vi "DataLog Databases Module.vi"(5 "LuaVIEW reference":T1, 7 "function index":i32) -> (15 "error out":errorcluster)   [LabVIEW 2012]
doc: "Module required by the \"databases\" runlevel. It enumerates the logging databases by scanning their directories and instantiates in-memory objects reflecting the tags in each database. Performs recovery of aggregated log data if needed. Exports tag management and query functions."
uses:
  luaview/typedefs/t_LuaVIEW Reference.ctl
  typedefs/t_DataLog Databases Methods.ctl
  typedefs/t_Datalog Datebase Modes.ctl
  typedefs/t_DataLog Tag Info List Methods.ctl
  luaview/subvis/private/LuaVIEW Pull (string).vi
  luaview/subvis/private/LuaVIEW Pull (refnum).vi
  subvis/private/glb_DataLog Runtime Parameterisation.vi
  luaview/subvis/private/LuaVIEW Pull (flat data).vi
  luaview/subvis/private/LuaVIEW Push (object).vi
  luaview/subvis/private/LuaVIEW Push (string).vi
  subvis/private/glb_DataLog MCVD.vi
  luaview/subvis/private/LuaVIEW Pull (number).vi
  luaview/subvis/private/LuaVIEW Push (boolean).vi
  luaview/subvis/private/LuaVIEW Push (flat data).vi
  luaview/subvis/private/LuaVIEW Push (number).vi
  luaview/subvis/private/LuaVIEW Push (I32).vi
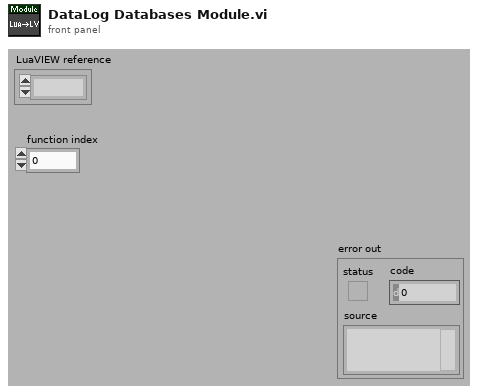
[diagram p1: front panel]
types:
  T1 = typedef "t_LuaVIEW Reference.ctl" = refnum<k1>
  T2 = enum32{"initialize", "init config", "init check config", "init recover", "init error?", "!DB.lookup([str:name])", "!DB.create(obj:db,str:tag,tab:config,[any:initial])", "!DB.delete(obj:db,str:tag)", "!bool:exists=DB.exists(obj:db,str:tag)", "!tab:config=DB.config(obj:db,str:tag)", "!tab:tags=DB.list(obj:db,[str:pattern])", "!any:value,num:time=DB.last(obj:db,str:tag)", "!num:values=DB.logsize(obj:db,str:tag)", "!str:mode=DB.mode(obj:db)", "!DB.reconfigure(obj:db,str:tag,tab:config)", "!tab:tags=DB.subset(obj:db,str:subset)", "!tab:subsets=DB.subsets(obj:db)", "!num:tags=DB.tags(obj:db)", "!str:basetag=stripmeta(str:metatag)", "revoke_exports()", "cleanup()"}
  T3 = typedef "t_DataLog Databases Methods.ctl" = enum16{"initialize", "get ref", "get names", "cleanup"}
  T4 = typedef "t_DataLog Tag Info List Methods.ctl" = enum16{"initialize", "create", "create empty", "rename", "delete", "test tag", "get", "get by name", "get default", "get list", "get path", "get subsets", "set subsets", "set config", "set capacity", "#tags", "go live", "set unlocked", "set mirrored"}
  T5 = typedef "t_Datalog Datebase Modes.ctl" = enum16{"locked", "unlocked", "live", "mirrored"}
  T6 = cluster{"databases":cluster{"mode":T5, "path":path}[], "recovery directory":path, "max points":i32, "max string mem":i32}
  T7 = typedef "t_DataLog Database Info Pane.ctl" = refnum<vi>
  T8 = typedef "t_DataLog Tag Config.ctl" = cluster{"name":string, "unit":string, "temporal":T9, "value":T10, "index":i32, "capacity":i32, "is meta?":bool, "mincapacity":i32, "deadband":dbl, "limit delay":dbl, "format":T11, "precision":u8, "undefine":bool, "update":bool, "update period":u16, "expression":string, "description":string, "logging algorithm":T12, "logging parameters":dbl[]}
  T9 = typedef "t_DataLog Temporal Types.ctl" = enum16{"set&hold", "sample", "event"}
  T10 = typedef "t_DataLog Value Types.ctl" = enum16{"number", "string"}
  T11 = typedef "t_DataLog Numerical Format.ctl" = enum8{"fractional", "exponential", "engineering"}
  T12 = typedef "t_DataLog Logging Algorithms.ctl" = enum16{"nothing", "changes", "everything", "every Nth", "time threshold", "value threshold + prior", "t or v threshold", "t or v threshold + prior"}
  T13 = typedef "et_DataLog Meta Tag Specifier.ctl" = enum32{"warn_lo", "warn_hi", "A_lo", "A_hi", "B_lo", "B_hi", "C_lo", "C_hi", "D_lo", "D_hi", "E_lo", "E_hi", "F_lo", "F_hi", "G_lo", "G_hi", "H_lo", "H_hi", "I_lo", "I_hi", "J_lo", "J_hi", "K_lo", "K_hi", "L_lo", "L_hi", "M_lo", "M_hi", "N_lo", "N_hi", "min", "max", "not a meta"}
  T14 = typedef "t_DataLog Point.ctl" = cluster{"time":dbl, "value":dbl}
  T15 = typedef "t_DataLog Tag Subset.ctl" = cluster{"name":string, "tags":string[]}
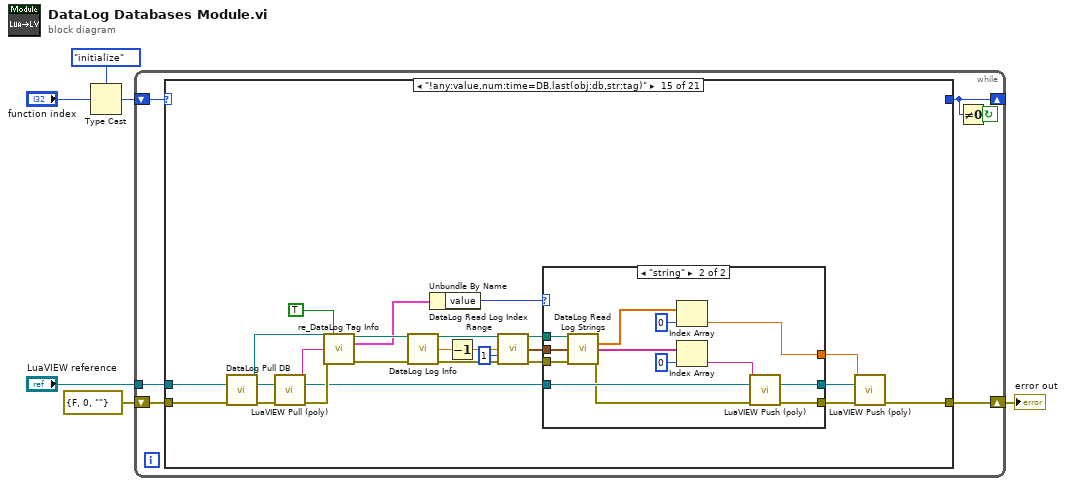
[diagram p0: block diagram]
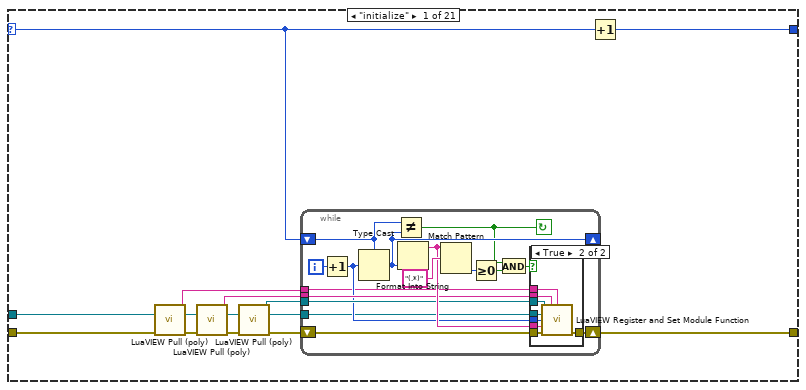
[diagram p2: hidden frame]
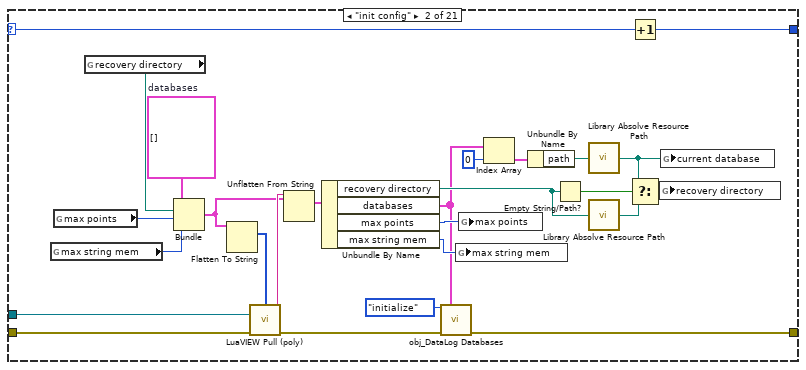
[diagram p4: hidden frame]
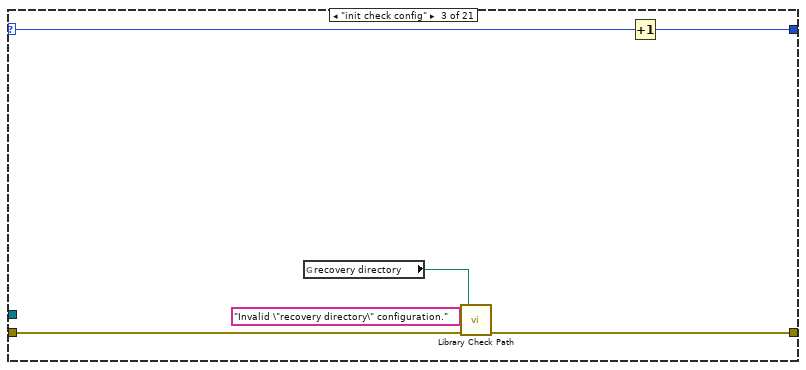
[diagram p5: hidden frame]
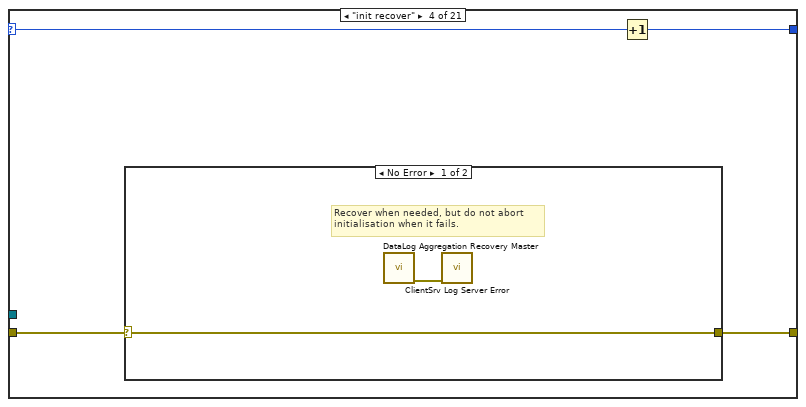
[diagram p6: hidden frame]
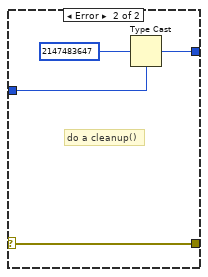
[diagram p9: hidden frame]
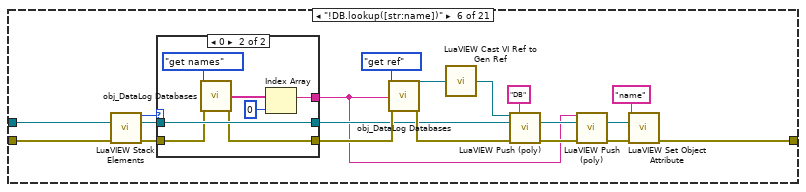
[diagram p10: hidden frame]
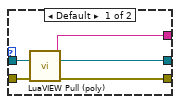
[diagram p11: hidden frame]
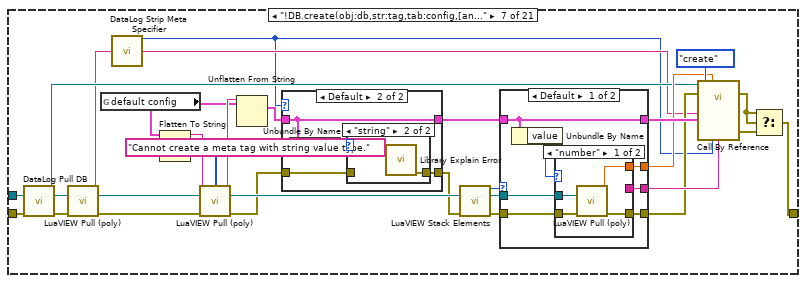
[diagram p12: hidden frame]
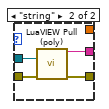
[diagram p15: hidden frame]
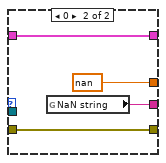
[diagram p16: hidden frame]
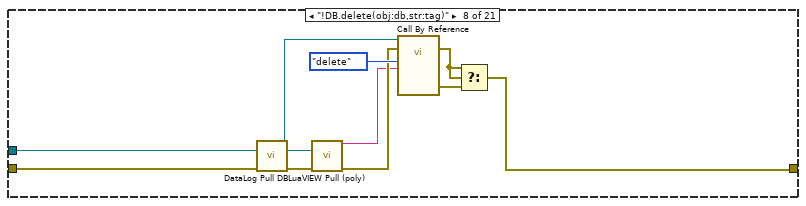
[diagram p17: hidden frame]
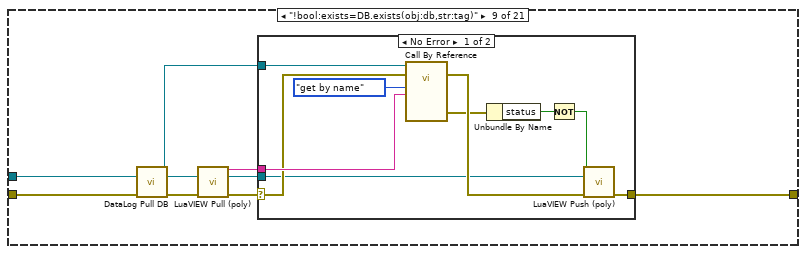
[diagram p18: hidden frame]
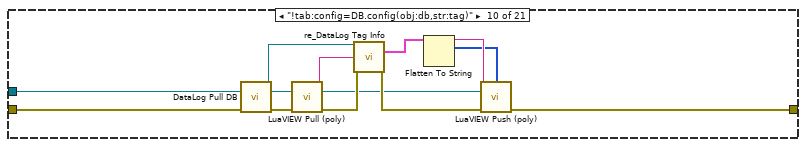
[diagram p20: hidden frame]
diagram:
  n1 = Type Cast(type=T2."initialize" ("cases"), x="function index") -> (*(type *) &x=w5:T2)
  n2 = while {
    shift-right: [w8] -> _
    shift-left: w5 -> [w12]
    shift-right: [w11] -> w6
    shift-left: errorcluster {"status"=FALSE, "code"=0, "source"=""} ("error out") -> [w10]
    tunnel: "LuaVIEW reference" -> [w9]
    stop <- w7 continue-if-true
    n3 = case shown="\"!any:value,num:time=DB.last(obj:db,str:tag)\"" w12 {
      selector: w12 -> [w14 w66 w80 w87 w94 _ _ _ _ _ _ _ _ _ _ _ _ _ _ _ _]
      tunnel: [w13 w67 w79 w86 w91 _ _ _ _ _ _ _ _ _ _ _ _ _ _ _ _] -> w8
      tunnel: w9 -> [w18 w75 _ _ _ w114 w144 w194 w207 w228 w249 w289 w301 w311 w332 w382 w429 w441 w449 w463 _]
      tunnel: [w26 w61 w81 w84 w92 w105 w159 w199 w205 w232 w241 w286 w298 w320 w335 w379 w425 w438 w446 w464 w467] -> w11
      tunnel: w10 -> [w17 w74 w78 w85 w93 w118 w145 w195 w208 w229 w248 w290 w302 w312 w333 w381 w428 w442 w450 w465 w467]
      frame "initialize" {
        n4 = call-poly "LuaVIEW Pull (poly).vi"("LuaVIEW reference in"=w18, "error in (no error)"=w17) -> ("string"=w21:string, "LuaVIEW reference out"=w23:T1, "error out"=w22:errorcluster)  [unwired: 11 in]
        n5 = call-poly "LuaVIEW Pull (poly).vi"("LuaVIEW reference in"=w23, "error in (no error)"=w22) -> ("string"=w25:string, "LuaVIEW reference out"=w19:T1, "error out"=w20:errorcluster)  [unwired: 11 in]
        n6 = call-poly "LuaVIEW Pull (poly).vi"("LuaVIEW reference in"=w19, "error in (no error)"=w20) -> ("refnum"=w24:refnum<vi>, "LuaVIEW reference out"=w16:T1, "error out"=w15:errorcluster)  [unwired: 11 in]
        n7 = while {
          tunnel: w21 -> [w30]
          shift-right: [w39] -> w26
          shift-left: w15 -> [w40]
          shift-right: [w35] -> _
          shift-left: w14 -> [w36]
          tunnel: w25 -> [w33]
          tunnel: w16 -> [w31]
          tunnel: w24 -> [w34]
          i -> [w38]
          stop <- w27 continue-if-true
          n8 = Increment(x=w38) -> (x+1=w32:i32)
          n9 = Type Cast(type=w36, x=w32) -> (*(type *) &x=w35:T2)
          n10 = Not Equal?(x=w36, y=w35) -> (x != y?=w27:bool)
          n11 = Format Into String(w35) -> (resulting string=w37:string)  [unwired: 3 in, 1 out]
          n12 = Match Pattern(string=w37, regular expression="(.*)") -> (offset past match=w41:i32)  [unwired: 1 in, 3 out]
          n13 = Greater Or Equal To 0?(x=w41) -> (x >= 0?=w29:bool)
          n14 = And(x=w27, y=w29) -> (x .and. y?=w28:bool)
          n15 = case shown="True" w28 {
            tunnel: w30 -> [_ w45]
            tunnel: w31 -> [_ w49]
            tunnel: w32 -> [_ w50]
            tunnel: w37 -> [_ w47]
            tunnel: [w43 w51] -> w39
            tunnel: w40 -> [w43 w48]
            tunnel: w33 -> [_ w46]
            tunnel: w34 -> [_ w44]
            frame False {
            }
            frame True {
              n16 = call "LuaVIEW Register and Set Module Function.vi"("module refnum"=w44, "export table (set as global)"=w46, "table (set as global)"=w45, "LuaVIEW reference in"=w49, "index"=w50, "synopsis"=w47, "error in (no error)"=w48) -> ("error out"=w51:errorcluster)  [unwired: 7 in, 1 out]
            }
          }
        }
        n17 = Increment(x=w14) -> (x+1=w13:T2)
      }
      frame "init config" {
        w63 = cluster{"mode":T5, "path":path}[] []  # databases
        n18 = global read "glb_DataLog Runtime Parameterisation.vi" "max string mem"() -> (w54:i32)
        n19 = global read "glb_DataLog Runtime Parameterisation.vi" "max points"() -> (w57:i32)
        n20 = global read "glb_DataLog Runtime Parameterisation.vi" "recovery directory"() -> (w72:path)
        n21 = Bundle("databases"=w63, "recovery directory"=w72, "max points"=w57, "max string mem"=w54) -> (w73:T6)  [unwired: 1 in]
        n22 = Flatten To String(anything=w73) -> (type string=w77:i16[])  [unwired: 3 in, 2 out]
        n23 = call-poly "LuaVIEW Pull (poly).vi"("type descriptor"=w77, "LuaVIEW reference in"=w75, "error in (no error)"=w74) -> ("flat data"=w76:string, "error out"=w65:errorcluster)  [unwired: 10 in, 1 out]
        n24 = Unflatten From String(type=w73, binary string=w76) -> (value=w71:T6)  [unwired: 3 in, 2 out]
        n25 = Unbundle By Name(w71) -> ("recovery directory"=w64:path, "databases"=w52:cluster{"mode":T5, "path":path}[], "max points"=w56:i32, "max string mem"=w53:i32)
        n26 = call "obj_DataLog Databases.vi"("method"=t_DataLog_Databases_Methods."initialize", "databases config {initialize}"=w52, "error in (no error)"=w65) -> ("error out"=w61:errorcluster)  [unwired: 10 in, 2 out]
        n27 = global write "glb_DataLog Runtime Parameterisation.vi" "max string mem"(w53) -> ()
        n28 = global write "glb_DataLog Runtime Parameterisation.vi" "max points"(w56) -> ()
        n29 = Index Array(array=w52, index=0) -> (element=w60:cluster{"mode":T5, "path":path})
        n30 = Unbundle By Name(w60) -> ("path"=w59:path)
        n31 = Empty String/Path?(string/path=w64) -> (empty?=w70:bool)
        n32 = call "Library Absolve Resource Path.vi"("path in"=w59) -> ("absolved path"=w55:path)  [unwired: 14 in]
        n33 = call "Library Absolve Resource Path.vi"("path in"=w64) -> ("absolved path"=w69:path)  [unwired: 14 in]
        n34 = Increment(x=w66) -> (x+1=w67:T2)
        n35 = Select(t=w55, s=w70, f=w69) -> (s? t:f=w68:path)
        n36 = global write "glb_DataLog Runtime Parameterisation.vi" "recovery directory"(w68) -> ()
        n37 = global write "glb_DataLog Runtime Parameterisation.vi" "current database"(w55) -> ()
      }
      frame "init check config" {
        n38 = global read "glb_DataLog Runtime Parameterisation.vi" "recovery directory"() -> (w82:path)
        n39 = call "Library Check Path.vi"("error in (no error)"=w78, "further explanation (none)"="Invalid \"recovery directory\" configuration.", "path"=w82) -> ("error out"=w81:errorcluster)  [unwired: 3 in, 1 out]
        n40 = Increment(x=w80) -> (x+1=w79:T2)
      }
      frame "init recover" {
        n41 = case shown="No Error" w85 {
          selector: w85 -> [w89 w90]
          tunnel: [w89 w90] -> w84
          frame No Error {
            # "Recover when needed, but do not abort\ninitialisation when it fails."
            n42 = call "DataLog Aggregation Recovery Master.vi"() -> ("error out"=w88:errorcluster)  [unwired: 15 in]
            n43 = call "ClientSrv Log Server Error.vi"("error (use message)"=w88) -> ()  [unwired: 15 in]
          }
          frame Error {
          }
        }
        n44 = Increment(x=w87) -> (x+1=w86:T2)
      }
      frame "init error?" {
        n45 = case shown="No Error" w93 {
          selector: w93 -> [w95 w97]
          tunnel: w94 -> [_ w98]
          tunnel: [w95 w97] -> w92
          tunnel: [_ w96] -> w91
          frame No Error {
          }
          frame Error {
            # "do a cleanup()"
            n46 = Type Cast(type=w98, x=2147483647) -> (*(type *) &x=w96:T2)
          }
        }
      }
      frame "!DB.lookup([str:name])" {
        n47 = call "LuaVIEW Stack Elements.vi"("LuaVIEW reference in"=w114, "error in (no error)"=w118) -> ("elements"=w116:i32, "LuaVIEW reference out"=w115:T1, "error out"=w117:errorcluster)  [unwired: 11 in]
        n48 = case shown="0" w116 {
          tunnel: w117 -> [w123 w128]
          tunnel: w115 -> [w122 w130]
          tunnel: [w121 w130] -> w104
          tunnel: [w120 w124] -> w101
          tunnel: [w119 w127] -> w113
          frame Default {
            n49 = call-poly "LuaVIEW Pull (poly).vi"("LuaVIEW reference in"=w122, "error in (no error)"=w123) -> ("string"=w120:string, "LuaVIEW reference out"=w121:T1, "error out"=w119:errorcluster)  [unwired: 11 in]
          }
          frame 0 {
            n50 = call "obj_DataLog Databases.vi"("method"=t_DataLog_Databases_Methods."get names", "error in (no error)"=w128) -> ("database names"=w126:string[], "error out"=w127:errorcluster)  [unwired: 11 in, 1 out]
            n51 = Index Array(array=w126, index=0) -> (element=w124:string)
          }
        }
        n52 = call "obj_DataLog Databases.vi"("method"=t_DataLog_Databases_Methods."get ref", "database (current)"=w101, "error in (no error)"=w113) -> ("database ref"=w100:T7, "error out"=w111:errorcluster)  [unwired: 10 in, 1 out]
        n53 = call "LuaVIEW Cast VI Ref to Gen Ref.vi"("refnum in"=w100) -> ("refnum out"=w102:refnum<vi>)  [unwired: 14 in]
        n54 = call-poly "LuaVIEW Push (poly).vi"("object refnum"=w102, "method table (use caller's function table)"="DB", "LuaVIEW reference in"=w104, "error in (no error)"=w111) -> ("LuaVIEW reference out"=w103:T1, "error out"=w106:errorcluster)  [unwired: 10 in]
        n55 = call-poly "LuaVIEW Push (poly).vi"("string"=w101, "LuaVIEW reference in"=w103, "error in (no error)"=w106) -> ("LuaVIEW reference out"=w109:T1, "error out"=w108:errorcluster)  [unwired: 11 in]
        n56 = call "LuaVIEW Set Object Attribute.vi"("key"="name", "LuaVIEW reference in"=w109, "error in (no error)"=w108) -> ("error out"=w105:errorcluster)  [unwired: 11 in, 1 out]
      }
      frame "!DB.create(obj:db,str:tag,tab:config,[any:initial])" {
        n57 = call "DataLog Pull DB.vi"("LuaVIEW reference in"=w144, "error in (no error)"=w145) -> ("database info"=w143:T7, "LuaVIEW reference out"=w134:T1, "error out"=w135:errorcluster)  [unwired: 11 in]
        n58 = call-poly "LuaVIEW Pull (poly).vi"("LuaVIEW reference in"=w134, "error in (no error)"=w135) -> ("string"=w131:string, "LuaVIEW reference out"=w132:T1, "error out"=w133:errorcluster)  [unwired: 11 in]
        n59 = global read "glb_DataLog MCVD.vi" "default config"() -> (w146:T8)
        n60 = call "DataLog Strip Meta Specifier.vi"("tag"=w131) -> ("meta specifier"=w141:T13, "base tag"=w142:string)  [unwired: 13 in]
        n61 = Flatten To String(anything=w146) -> (data string=w158:string, type string=w157:i16[])  [unwired: 3 in, 1 out]
        n62 = call-poly "LuaVIEW Pull (poly).vi"("default flat data"=w158, "type descriptor"=w157, "LuaVIEW reference in"=w132, "error in (no error)"=w133) -> ("flat data"=w156:string, "LuaVIEW reference out"=w138:T1, "error out"=w137:errorcluster)  [unwired: 9 in]
        n63 = Unflatten From String(type=w146, binary string=w156) -> (value=w140:T8)  [unwired: 3 in, 2 out]
        n64 = case shown="Default" w141 {
          tunnel: w140 -> [w162 w165]
          tunnel: [w162 w165] -> w139
          tunnel: w137 -> [w161 w163]
          tunnel: [w161 w166] -> w136
          frame "not a meta" {
          }
          frame Default {
            n65 = Unbundle By Name(w165) -> ("value"=w164:T10)
            n66 = case shown="\"string\"" w164 {
              tunnel: [w167 w169] -> w166
              tunnel: w163 -> [w167 _]
              frame "number" {
              }
              frame "string" {
                n67 = call "Library Explain Error.vi"("explanation prefix (none)"="Cannot create a meta tag with string value type.") -> ("explained error"=w169:errorcluster)  [unwired: 14 in]
              }
            }
          }
        }
        n68 = call "LuaVIEW Stack Elements.vi"("LuaVIEW reference in"=w138, "error in (no error)"=w136) -> ("elements"=w153:i32, "LuaVIEW reference out"=w149:T1, "error out"=w148:errorcluster)  [unwired: 11 in]
        n69 = case shown="Default" w153 {
          tunnel: w139 -> [w176 w188]
          tunnel: [w176 w188] -> w152
          tunnel: [w170 nan] -> w151
          tunnel: [w171 w185] -> w150
          tunnel: w149 -> [w172 _]
          tunnel: [w173 w186] -> w147
          tunnel: w148 -> [w174 w186]
          frame Default {
            n70 = Unbundle By Name(w176) -> ("value"=w175:T10)
            n71 = case shown="\"number\"" w175 {
              tunnel: w174 -> [w180 w184]
              tunnel: [w179 w183] -> w173
              tunnel: w172 -> [w178 w182]
              tunnel: [_ w181] -> w171
              tunnel: [w177 _] -> w170
              frame "number" {
                n72 = call-poly "LuaVIEW Pull (poly).vi"("LuaVIEW reference in"=w178, "error in (no error)"=w180) -> ("number"=w177:dbl, "error out"=w179:errorcluster)  [unwired: 11 in, 1 out]
              }
              frame "string" {
                n73 = call-poly "LuaVIEW Pull (poly).vi"("LuaVIEW reference in"=w182, "error in (no error)"=w184) -> ("string"=w181:string, "error out"=w183:errorcluster)  [unwired: 11 in, 1 out]
              }
            }
          }
          frame 0 {
            n74 = global read "glb_DataLog MCVD.vi" "NaN string"() -> (w185:string)
          }
        }
        n75 = call-by-ref "?"(reference=w143, error in=w147, "method"=t_DataLog_Tag_Info_List_Methods."create", "initial number (NaN)"=w151, "tag or base tag"=w142, "tag config in"=w152, "meta specifier (not a meta)"=w141, "initial string (\"\")"=w150) -> (error out=w154:errorcluster, 15:"error out"=w155:errorcluster)  [unwired: 3 in, 7 out]
        n76 = Select(t=w154, s=w154, f=w155) -> (s? t:f=w159:errorcluster)
      }
      frame "!DB.delete(obj:db,str:tag)" {
        n77 = call "DataLog Pull DB.vi"("LuaVIEW reference in"=w194, "error in (no error)"=w195) -> ("database info"=w193:T7, "LuaVIEW reference out"=w189:T1, "error out"=w192:errorcluster)  [unwired: 11 in]
        n78 = call-poly "LuaVIEW Pull (poly).vi"("LuaVIEW reference in"=w189, "error in (no error)"=w192) -> ("string"=w190:string, "error out"=w191:errorcluster)  [unwired: 11 in, 1 out]
        n79 = call-by-ref "?"(reference=w193, error in=w191, "method"=t_DataLog_Tag_Info_List_Methods."delete", "tag or base tag"=w190) -> (error out=w196:errorcluster, 15:"error out"=w197:errorcluster)  [unwired: 7 in, 7 out]
        n80 = Select(t=w196, s=w196, f=w197) -> (s? t:f=w199:errorcluster)
      }
      frame "!bool:exists=DB.exists(obj:db,str:tag)" {
        n81 = call "DataLog Pull DB.vi"("LuaVIEW reference in"=w207, "error in (no error)"=w208) -> ("database info"=w206:T7, "LuaVIEW reference out"=w204:T1, "error out"=w203:errorcluster)  [unwired: 11 in]
        n82 = call-poly "LuaVIEW Pull (poly).vi"("LuaVIEW reference in"=w204, "error in (no error)"=w203) -> ("string"=w200:string, "LuaVIEW reference out"=w202:T1, "error out"=w201:errorcluster)  [unwired: 11 in]
        n83 = case shown="No Error" w201 {
          selector: w201 -> [w215 w219]
          tunnel: w206 -> [w217 _]
          tunnel: w200 -> [w216 _]
          tunnel: [w212 w219] -> w205
          tunnel: w202 -> [w211 _]
          frame No Error {
            n84 = call-by-ref "?"(reference=w217, error in=w215, "method"=t_DataLog_Tag_Info_List_Methods."get by name", "tag or base tag"=w216) -> (error out=w214:errorcluster, 15:"error out"=w213:errorcluster)  [unwired: 7 in, 7 out]
            n85 = Unbundle By Name(w213) -> ("status"=w210:bool)
            n86 = Not(x=w210) -> (.not. x?=w209:bool)
            n87 = call-poly "LuaVIEW Push (poly).vi"("boolean"=w209, "LuaVIEW reference in"=w211, "error in (no error)"=w214) -> ("error out"=w212:errorcluster)  [unwired: 11 in, 1 out]
          }
          frame Error {
          }
        }
      }
      frame "!tab:config=DB.config(obj:db,str:tag)" {
        n88 = call "DataLog Pull DB.vi"("LuaVIEW reference in"=w228, "error in (no error)"=w229) -> ("database info"=w227:T7, "LuaVIEW reference out"=w223:T1, "error out"=w224:errorcluster)  [unwired: 11 in]
        n89 = call-poly "LuaVIEW Pull (poly).vi"("LuaVIEW reference in"=w223, "error in (no error)"=w224) -> ("string"=w221:string, "LuaVIEW reference out"=w220:T1, "error out"=w222:errorcluster)  [unwired: 11 in]
        n90 = call "re_DataLog Tag Info.vi"("database ref (use name)"=w227, "tag"=w221, "error in (no error)"=w222) -> ("tag config"=w225:T8, "error out"=w226:errorcluster)  [unwired: 9 in, 2 out]
        n91 = Flatten To String(anything=w225) -> (data string=w231:string, type string=w230:i16[])  [unwired: 3 in, 1 out]
        n92 = call-poly "LuaVIEW Push (poly).vi"("flat data"=w231, "type descriptor"=w230, "LuaVIEW reference in"=w220, "error in (no error)"=w226) -> ("error out"=w232:errorcluster)  [unwired: 10 in, 1 out]
      }
      frame "!tab:tags=DB.list(obj:db,[str:pattern])" {
        n93 = call "DataLog Pull DB.vi"("LuaVIEW reference in"=w249, "error in (no error)"=w248) -> ("database info"=w233:T7, "LuaVIEW reference out"=w247:T1, "error out"=w246:errorcluster)  [unwired: 11 in]
        n94 = call-by-ref "?"(reference=w233, error in=w246, "method"=t_DataLog_Tag_Info_List_Methods."get list") -> (error out=w234:errorcluster, "tag config list"=w243:T8[], 15:"error out"=w235:errorcluster)  [unwired: 8 in, 6 out]
        n95 = for {
          tunnel: w243 -> [w254] mode=indexing
          tunnel: [w253] -> w242 mode=indexing
          n96 = Unbundle By Name(w254) -> ("name"=w253:string)
        }
        n97 = Select(t=w234, s=w234, f=w235) -> (s? t:f=w244:errorcluster)
        n98 = call "LuaVIEW Stack Elements.vi"("LuaVIEW reference in"=w247, "error in (no error)"=w244) -> ("elements"=w251:i32, "LuaVIEW reference out"=w250:T1, "error out"=w252:errorcluster)  [unwired: 11 in]
        n99 = case shown="Default" w251 {
          tunnel: w252 -> [w263 w275]
          tunnel: w250 -> [w262 w276]
          tunnel: [w258 w276] -> w240
          tunnel: [w260 w274] -> w239
          tunnel: [w257 w275] -> w238
          tunnel: w242 -> [w261 w274]
          frame Default {
            n100 = call-poly "LuaVIEW Pull (poly).vi"("LuaVIEW reference in"=w262, "error in (no error)"=w263) -> ("string"=w259:string, "LuaVIEW reference out"=w258:T1, "error out"=w257:errorcluster)  [unwired: 11 in]
            n101 = call "Library Wildcards to Regular.vi"("wildcards"=w259) -> ("regular expression"=w255:string)  [unwired: 4 in]
            n102 = for {
              tunnel: w261 -> [w265] mode=indexing
              shift-right: [w268] -> w260
              shift-left: string[] [] -> [w269]
              tunnel: w255 -> [w267]
              n103 = Match Pattern(string=w265, regular expression=w267) -> (offset past match=w266:i32)  [unwired: 1 in, 3 out]
              n104 = Greater Or Equal To 0?(x=w266) -> (x >= 0?=w264:bool)
              n105 = case shown="True" w264 {
                tunnel: w269 -> [w270 w273]
                tunnel: [w270 w272] -> w268
                tunnel: w265 -> [_ w271]
                frame False {
                }
                frame True {
                  n106 = Build Array (concatenate)(w273, w271) -> (w272:string[])
                }
              }
            }
          }
          frame 0 {
          }
        }
        n107 = Flatten To String(anything=w239) -> (data string=w236:string, type string=w237:i16[])  [unwired: 3 in, 1 out]
        n108 = call-poly "LuaVIEW Push (poly).vi"("flat data"=w236, "type descriptor"=w237, "LuaVIEW reference in"=w240, "error in (no error)"=w238) -> ("error out"=w241:errorcluster)  [unwired: 10 in, 1 out]
      }
      frame "!num:values=DB.logsize(obj:db,str:tag)" {
        n109 = call "DataLog Pull DB.vi"("LuaVIEW reference in"=w289, "error in (no error)"=w290) -> ("database info"=w284:T7, "LuaVIEW reference out"=w280:T1, "error out"=w281:errorcluster)  [unwired: 11 in]
        n110 = call-poly "LuaVIEW Pull (poly).vi"("LuaVIEW reference in"=w280, "error in (no error)"=w281) -> ("string"=w277:string, "LuaVIEW reference out"=w279:T1, "error out"=w278:errorcluster)  [unwired: 11 in]
        n111 = call "re_DataLog Tag Info.vi"("database ref (use name)"=w284, "flush? (false)"=TRUE, "tag"=w277, "error in (no error)"=w278) -> ("tag log directory"=w282:path, "error out"=w285:errorcluster)  [unwired: 8 in, 2 out]
        n112 = call "DataLog Log Info.vi"("tag log directory"=w282, "error in (no error)"=w285) -> ("size"=w287:dbl, "error out"=w288:errorcluster)  [unwired: 10 in, 2 out]
        n113 = call-poly "LuaVIEW Push (poly).vi"("number"=w287, "LuaVIEW reference in"=w279, "error in (no error)"=w288) -> ("error out"=w286:errorcluster)  [unwired: 11 in, 1 out]
      }
      frame "!str:mode=DB.mode(obj:db)" {
        n114 = call "DataLog Pull DB.vi"("LuaVIEW reference in"=w301, "error in (no error)"=w302) -> ("database info"=w300:T7, "LuaVIEW reference out"=w297:T1, "error out"=w299:errorcluster)  [unwired: 11 in]
        n115 = call-by-ref "?"(reference=w300, error in=w299, "method"=t_DataLog_Tag_Info_List_Methods."#tags") -> (error out=w295:errorcluster, "mode"=w292:T5, 15:"error out"=w294:errorcluster)  [unwired: 8 in, 6 out]
        n116 = Select(t=w295, s=w295, f=w294) -> (s? t:f=w293:errorcluster)
        n117 = Format Into String(w292) -> (resulting string=w291:string)  [unwired: 3 in, 1 out]
        n118 = call-poly "LuaVIEW Push (poly).vi"("string"=w291, "LuaVIEW reference in"=w297, "error in (no error)"=w293) -> ("error out"=w298:errorcluster)  [unwired: 11 in, 1 out]
      }
      frame "!DB.reconfigure(obj:db,str:tag,tab:config)" {
        n119 = call "DataLog Pull DB.vi"("LuaVIEW reference in"=w311, "error in (no error)"=w312) -> ("database info"=w310:T7, "LuaVIEW reference out"=w306:T1, "error out"=w307:errorcluster)  [unwired: 11 in]
        n120 = call-poly "LuaVIEW Pull (poly).vi"("LuaVIEW reference in"=w306, "error in (no error)"=w307) -> ("string"=w303:string, "LuaVIEW reference out"=w305:T1, "error out"=w304:errorcluster)  [unwired: 11 in]
        n121 = call "re_DataLog Tag Info.vi"("database ref (use name)"=w310, "tag"=w303, "error in (no error)"=w304) -> ("tag config"=w309:T8, "error out"=w308:errorcluster)  [unwired: 9 in, 2 out]
        n122 = Flatten To String(anything=w309) -> (data string=w319:string, type string=w318:i16[])  [unwired: 3 in, 1 out]
        n123 = call-poly "LuaVIEW Pull (poly).vi"("default flat data"=w319, "type descriptor"=w318, "LuaVIEW reference in"=w305, "error in (no error)"=w308) -> ("flat data"=w317:string, "error out"=w315:errorcluster)  [unwired: 9 in, 1 out]
        n124 = Unflatten From String(type=w309, binary string=w317) -> (value=w316:T8)  [unwired: 3 in, 2 out]
        n125 = call-by-ref "?"(reference=w310, error in=w315, "method"=t_DataLog_Tag_Info_List_Methods."set config", "tag or base tag"=w303, "tag config in"=w316) -> (error out=w313:errorcluster, 15:"error out"=w314:errorcluster)  [unwired: 6 in, 7 out]
        n126 = Select(t=w313, s=w313, f=w314) -> (s? t:f=w320:errorcluster)
      }
      frame "!any:value,num:time=DB.last(obj:db,str:tag)" {
        n127 = call "DataLog Pull DB.vi"("LuaVIEW reference in"=w332, "error in (no error)"=w333) -> ("database info"=w328:T7, "LuaVIEW reference out"=w325:T1, "error out"=w326:errorcluster)  [unwired: 11 in]
        n128 = call-poly "LuaVIEW Pull (poly).vi"("LuaVIEW reference in"=w325, "error in (no error)"=w326) -> ("string"=w322:string, "LuaVIEW reference out"=w323:T1, "error out"=w324:errorcluster)  [unwired: 11 in]
        n129 = call "re_DataLog Tag Info.vi"("database ref (use name)"=w328, "flush? (false)"=TRUE, "tag"=w322, "error in (no error)"=w324) -> ("tag log directory"=w331:path, "tag config"=w330:T8, "error out"=w329:errorcluster)  [unwired: 8 in, 1 out]
        n130 = call "DataLog Log Info.vi"("tag log directory"=w331, "error in (no error)"=w329) -> ("dup tag log directory"=w334:path, "size"=w342:dbl, "error out"=w339:errorcluster)  [unwired: 10 in, 1 out]
        n131 = Unbundle By Name(w330) -> ("value"=w346:T10)
        n132 = Decrement(x=w342) -> (x-1=w341:dbl)
        n133 = call "DataLog Read Log Index Range.vi"("tag log directory"=w334, "log index"=w341, "number of points"=1, "error in (no error)"=w339) -> ("dup tag log directory"=w345:path, "range of points"=w344:T14[], "error out"=w343:errorcluster)  [unwired: 9 in]
        n134 = case shown="\"string\"" w346 {
          tunnel: w343 -> [w355 w368]
          tunnel: w344 -> [w353 w367]
          tunnel: w345 -> [_ w366]
          tunnel: w323 -> [w354 w358]
          tunnel: [w349 w360] -> w338
          tunnel: [w348 w364] -> w337
          tunnel: [w347 w359] -> w336
          frame "number" {
            n135 = Index Array(array=w353, index=0) -> (element=w351:T14)
            n136 = Unbundle By Name(w351) -> ("time"=w348:dbl, "value"=w350:dbl)
            n137 = call-poly "LuaVIEW Push (poly).vi"("number"=w350, "LuaVIEW reference in"=w354, "error in (no error)"=w355) -> ("LuaVIEW reference out"=w347:T1, "error out"=w349:errorcluster)  [unwired: 11 in]
          }
          frame "string" {
            n138 = call "DataLog Read Log Strings.vi"("tag log directory"=w366, "points (use offsets)"=w367, "error in (no error)"=w368) -> ("times"=w365:dbl[], "strings"=w362:string[], "error out"=w357:errorcluster)  [unwired: 9 in, 1 out]
            n139 = Index Array(array=w365, index=0) -> (element=w364:dbl)
            n140 = Index Array(array=w362, index=0) -> (element=w356:string)
            n141 = call-poly "LuaVIEW Push (poly).vi"("string"=w356, "LuaVIEW reference in"=w358, "error in (no error)"=w357) -> ("LuaVIEW reference out"=w359:T1, "error out"=w360:errorcluster)  [unwired: 11 in]
          }
        }
        n142 = call-poly "LuaVIEW Push (poly).vi"("number"=w337, "LuaVIEW reference in"=w336, "error in (no error)"=w338) -> ("error out"=w335:errorcluster)  [unwired: 11 in, 1 out]
      }
      frame "!tab:tags=DB.subset(obj:db,str:subset)" {
        n143 = call "DataLog Pull DB.vi"("LuaVIEW reference in"=w382, "error in (no error)"=w381) -> ("database info"=w376:T7, "LuaVIEW reference out"=w373:T1, "error out"=w374:errorcluster)  [unwired: 11 in]
        n144 = call-poly "LuaVIEW Pull (poly).vi"("LuaVIEW reference in"=w373, "error in (no error)"=w374) -> ("string"=w370:string, "LuaVIEW reference out"=w371:T1, "error out"=w372:errorcluster)  [unwired: 11 in]
        n145 = call-by-ref "?"(reference=w376, error in=w372, "method"=t_DataLog_Tag_Info_List_Methods."get subsets") -> (error out=w377:errorcluster, "subsets out"=w375:T15[], 15:"error out"=w378:errorcluster)  [unwired: 8 in, 6 out]
        n146 = Select(t=w377, s=w377, f=w378) -> (s? t:f=w369:errorcluster)
        n147 = case shown="No Error" w369 {
          selector: w369 -> [w384 w415]
          tunnel: [w391 w415] -> w379
          tunnel: w375 -> [w390 _]
          tunnel: w371 -> [w389 _]
          tunnel: w370 -> [w383 _]
          frame No Error {
            n148 = for {
              tunnel: w390 -> [w410] mode=indexing
              tunnel: w383 -> [w408]
              shift-right: [w406] -> w386
              shift-left: string[] [] ("tags") -> [w404]
              shift-right: [w402] -> w385
              shift-left: FALSE -> [w403]
              n149 = Unbundle By Name(w410) -> ("name"=w409:string, "tags"=w405:string[])
              n150 = Equal?(x=w408, y=w409) -> (x = y?=w407:bool)
              n151 = case shown="True" w407 {
                tunnel: [w411 w414] -> w406
                tunnel: w405 -> [_ w414]
                tunnel: w404 -> [w411 _]
                tunnel: w403 -> [w412 _]
                tunnel: [w412 TRUE] -> w402
                frame False {
                }
                frame True {
                }
              }
            }
            n152 = case "subset found?" shown="False" w385 {
              tunnel: [w395 w401] -> w391
              tunnel: w384 -> [_ w398]
              tunnel: w389 -> [_ w397]
              tunnel: w386 -> [_ w396]
              tunnel: w383 -> [w393 _]
              frame False {
                n153 = Format Into String(format string="Specified tag subset \"%s\" does not exist" ("explanation prefix (none)"), w393) -> (resulting string=w392:string)  [unwired: 2 in, 1 out]
                n154 = call "Library Explain Error.vi"("explanation prefix (none)"=w392) -> ("explained error"=w395:errorcluster)  [unwired: 14 in]
              }
              frame True {
                n155 = Flatten To String(anything=w396) -> (data string=w399:string, type string=w400:i16[])  [unwired: 3 in, 1 out]
                n156 = call-poly "LuaVIEW Push (poly).vi"("flat data"=w399, "type descriptor"=w400, "LuaVIEW reference in"=w397, "error in (no error)"=w398) -> ("error out"=w401:errorcluster)  [unwired: 10 in, 1 out]
              }
            }
          }
          frame Error {
          }
        }
      }
      frame "!tab:subsets=DB.subsets(obj:db)" {
        n157 = call "DataLog Pull DB.vi"("LuaVIEW reference in"=w429, "error in (no error)"=w428) -> ("database info"=w420:T7, "LuaVIEW reference out"=w417:T1, "error out"=w427:errorcluster)  [unwired: 11 in]
        n158 = call-by-ref "?"(reference=w420, error in=w427, "method"=t_DataLog_Tag_Info_List_Methods."get subsets") -> (error out=w421:errorcluster, "subsets out"=w419:T15[], 15:"error out"=w422:errorcluster)  [unwired: 8 in, 6 out]
        n159 = Select(t=w421, s=w421, f=w422) -> (s? t:f=w416:errorcluster)
        n160 = for {
          tunnel: w419 -> [w431] mode=indexing
          tunnel: [w430] -> w418 mode=indexing
          n161 = Unbundle By Name(w431) -> ("name"=w430:string)
        }
        n162 = Flatten To String(anything=w418) -> (data string=w423:string, type string=w424:i16[])  [unwired: 3 in, 1 out]
        n163 = call-poly "LuaVIEW Push (poly).vi"("flat data"=w423, "type descriptor"=w424, "LuaVIEW reference in"=w417, "error in (no error)"=w416) -> ("error out"=w425:errorcluster)  [unwired: 10 in, 1 out]
      }
      frame "!num:tags=DB.tags(obj:db)" {
        n164 = call "DataLog Pull DB.vi"("LuaVIEW reference in"=w441, "error in (no error)"=w442) -> ("database info"=w440:T7, "LuaVIEW reference out"=w437:T1, "error out"=w439:errorcluster)  [unwired: 11 in]
        n165 = call-by-ref "?"(reference=w440, error in=w439, "method"=t_DataLog_Tag_Info_List_Methods."#tags") -> (error out=w435:errorcluster, "#tags/change#"=w432:i32, 15:"error out"=w434:errorcluster)  [unwired: 8 in, 6 out]
        n166 = Select(t=w435, s=w435, f=w434) -> (s? t:f=w433:errorcluster)
        n167 = call-poly "LuaVIEW Push (poly).vi"("I32"=w432, "LuaVIEW reference in"=w437, "error in (no error)"=w433) -> ("error out"=w438:errorcluster)  [unwired: 11 in, 1 out]
      }
      frame "!str:basetag=stripmeta(str:metatag)" {
        n168 = call-poly "LuaVIEW Pull (poly).vi"("LuaVIEW reference in"=w449, "error in (no error)"=w450) -> ("string"=w448:string, "LuaVIEW reference out"=w444:T1, "error out"=w447:errorcluster)  [unwired: 11 in]
        n169 = call "DataLog Strip Meta Specifier.vi"("tag"=w448) -> ("meta specifier"=w443:T13, "base tag"=w445:string)  [unwired: 13 in]
        n170 = case shown="Default" w443 {
          selector: w443 -> [_ w456]
          tunnel: w447 -> [_ w462]
          tunnel: [w454 w457] -> w446
          tunnel: w445 -> [w453 w461]
          tunnel: w444 -> [_ w460]
          frame "not a meta" {
            n171 = Format Into String(format string="\"%s\" is not a meta tag", w453) -> (resulting string=w451:string)  [unwired: 2 in, 1 out]
            n172 = call "Library Explain Error.vi"("explanation prefix (none)"=w451) -> ("explained error"=w454:errorcluster)  [unwired: 14 in]
          }
          frame Default {
            n173 = call-poly "LuaVIEW Push (poly).vi"("string"=w461, "LuaVIEW reference in"=w460, "error in (no error)"=w462) -> ("LuaVIEW reference out"=w458:T1, "error out"=w459:errorcluster)  [unwired: 11 in]
            n174 = Format Into String(w456) -> (resulting string=w455:string)  [unwired: 3 in, 1 out]
            n175 = call-poly "LuaVIEW Push (poly).vi"("string"=w455, "LuaVIEW reference in"=w458, "error in (no error)"=w459) -> ("error out"=w457:errorcluster)  [unwired: 11 in, 1 out]
          }
        }
      }
      frame "revoke_exports()" {
        n176 = call "LuaVIEW Revoke Exports.vi"("LuaVIEW reference in"=w463, "error in (no error)"=w465) -> ("error out"=w464:errorcluster)  [unwired: 12 in, 1 out]
      }
      frame "cleanup()" {
        n177 = call "obj_DataLog Databases.vi"("method"=t_DataLog_Databases_Methods."cleanup") -> ()  [unwired: 12 in, 3 out]
      }
    }
    n178 = Not Equal To 0?(x=w8) -> (x != 0?=w7:bool)
  }
  "error out" <- w6
